vi "MPXsetAmplitudeDC.vi"(1 "Amplitude [V]":i32=100, 2 "MPX COM-Port":refnum<visa-resource-name>="COM5") -> (0 "MPX COM-Port dup":refnum<visa-resource-name>="COM5")   [LabVIEW 2015]
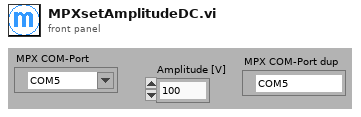
[diagram p1: front panel]
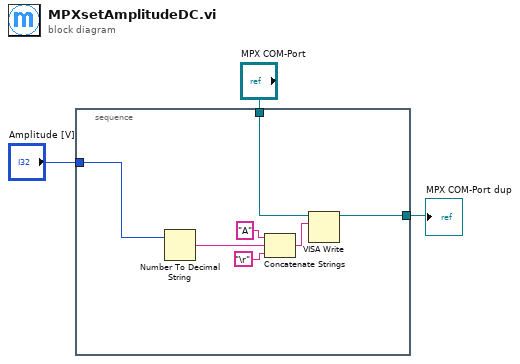
[diagram p0: block diagram]
diagram:
  n1 = stacked-sequence {
    tunnel: "MPX COM-Port" -> [w7]
    tunnel: "Amplitude [V]" -> [w6]
    tunnel: [w4] -> w1
    frame #0 {
      n2 = Number To Decimal String(number=w6) -> (decimal integer string=w5:string)  [unwired: 1 in]
      n3 = Concatenate Strings("A", w5, "\r") -> (w10:string)
      n4 = VISA Write(VISA resource name=w7, write buffer=w10) -> (VISA resource name out=w4:refnum<visa-resource-name>)  [unwired: 1 in, 2 out]
    }
  }
  "MPX COM-Port dup" <- w1
